vi "Global_ACT_Data Out.vi"() -> ()   [LabVIEW 2023, in "2024 Elevator_ACT.lvlib"]
uses:
  startup.rtexe/2024 Elevator_ACT.lvlib
  startup.rtexe/WPI_SolenoidValue.ctl
panel:
  in  "Lift Output":T1=enum."Forward"
  out "Compressor Running":bool
  out "Enabled":bool
  in  "ACT_Elevator_CycleTime(S)":dbl
  # "The Names of the Data items in the Global Variable MUST describe who the Single Writer is\nFor Actuator Globals the the naming convention is\n   \nACT_Lib Name_Data Name\n\nExamples:\nACT_Drive_X axis\nACT_Hopper_AgitatorSpeed"
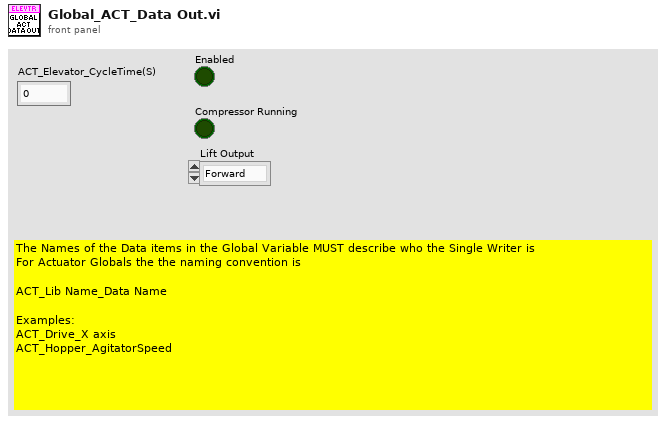
[diagram p1: front panel]
types:
  T1 = typedef "WPI_SolenoidValue.ctl" = enum16{"Off", "On", "Forward", "Reverse"}
diagram:
